vi "1D Look-Up Table (DBL Array).vi"(2 "LUT":dbl[](array[numeric]) format="%.2f", 3 "Indices":dbl[](array[numeric]) format="%.2f") -> (1 "Output Points":dbl[](array[numeric]) format="%.2f")   [LabVIEW 2020, in "NI_AdvCtrl_nonlinear.lvlib"]
doc: "LabVIEW no longer supports this VI. You can obtain similar functionality by installing the LabVIEW Simulation Module.\n\nSearches for an element in a given 1D list that has a fractional index (interpolation)."
uses:
  <vilib>/addons/control/advanced/NI_AdvCtrl_nonlinear.lvlib
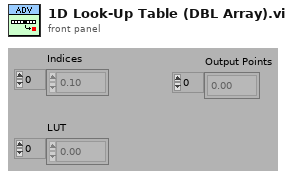
[diagram p1: front panel]
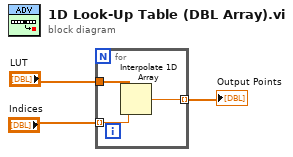
[diagram p0: block diagram]
diagram:
  n1 = for {
    tunnel: "Indices" -> [w6] mode=indexing
    tunnel: "LUT" -> [w5]
    tunnel: [w4] -> w1 mode=indexing
    n2 = Interpolate 1D Array(1:w6, 2:w5) -> (0:w4:dbl)
  }
  "Output Points" <- w1
